vi "Starast.vi"(4 "Ry":i32, 6 "Rx":i32, 8 "Centre Y":i32, 9 "Centre X":i32, 11 "Table Astrometry IN":T1 {"LONGPOLE" format="%.1f"}) -> (3 "Table Astrometry OUT":T1 {"LONGPOLE" format="%.1f"})   [LabVIEW 2019]
uses:
  Globals.vi
panel:
  in  "remove":bool
  in  "add":bool
  in  "Y":i32
  in  "X":i32
  in  "DEC":dbl format="%<%H:%M:%S>t"
  in  "RA":dbl format="%<%H:%M:%S%1u>t"
  in  "calcul":bool
  in  "cancel":bool
  in  "data":string[][](table) caption="Données Astrométriques"
  # "Cette routine permet de recalculer les paramètres du champ et des tables de \nguidage.  Pour ce faire, il faut qu'il y ait 2 ou 3 lignes de données astrométriques.\n\nRemplissez le tableau en centrant une étoile brillante dont la position est connue\nprès du centre optique, puis au moins une deuxième à plus de 15 minutes d'arc\ndu centre.  Idéalement, on voudra en enregistrer une 3e perpendiculairement\nà la deuxième et aussi éloignez d'au moins 15 minutes d'arc des deux autres.\n\nLorsque vous avez terminé, appuyer sur calculer pour voir le résultat du calcul \nou sur annuler pour ignorer tout ce qui a été fait ici."
  # "Voir la possibilité de faire le calcul sur\ntous les couples de 3 coordonnées ..."
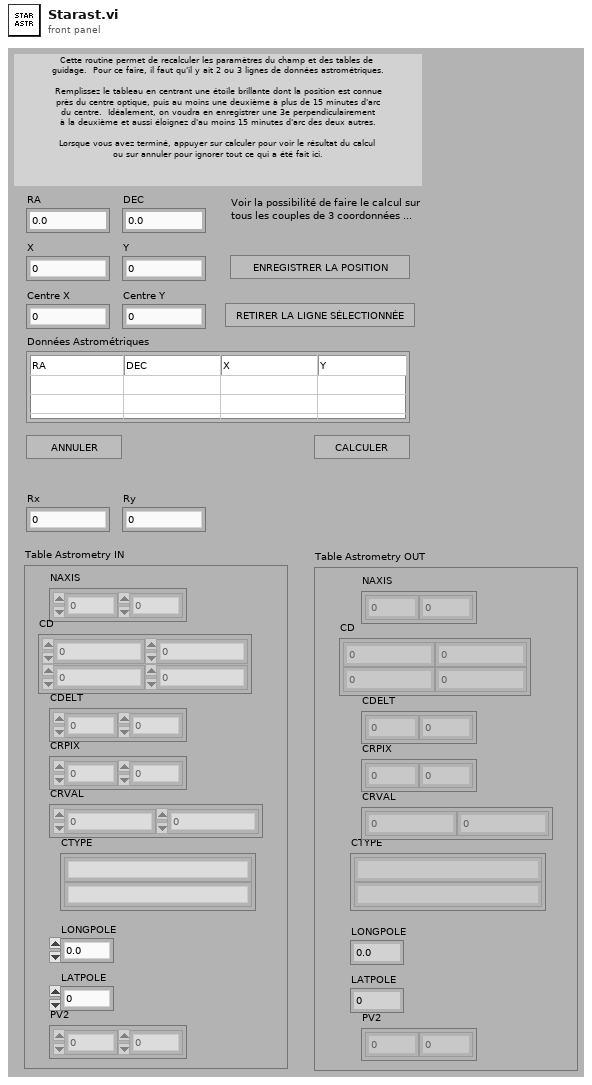
[diagram p1: front panel]
types:
  T1 = cluster{"NAXIS":dbl[], "CD":dbl[][], "CDELT":dbl[], "CRPIX":dbl[], "CTYPE":string[], "CRVAL":dbl[], "LONGPOLE":dbl, "LATPOLE":dbl, "PV2":dbl[]}
  T2 = typedef "LVRowAndColumnTypeDef.ctl" = cluster{"Row":i32, "Column":i32}
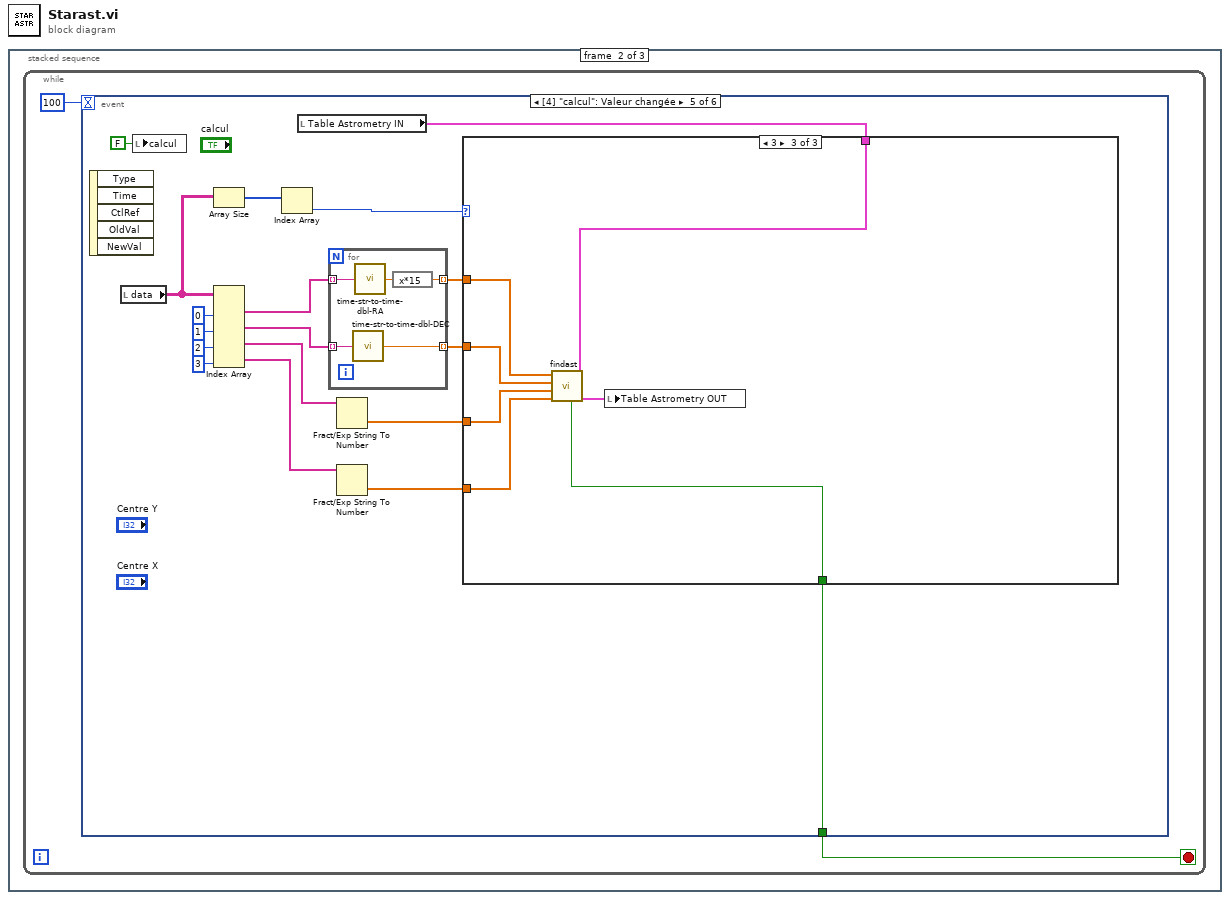
[diagram p0: block diagram]
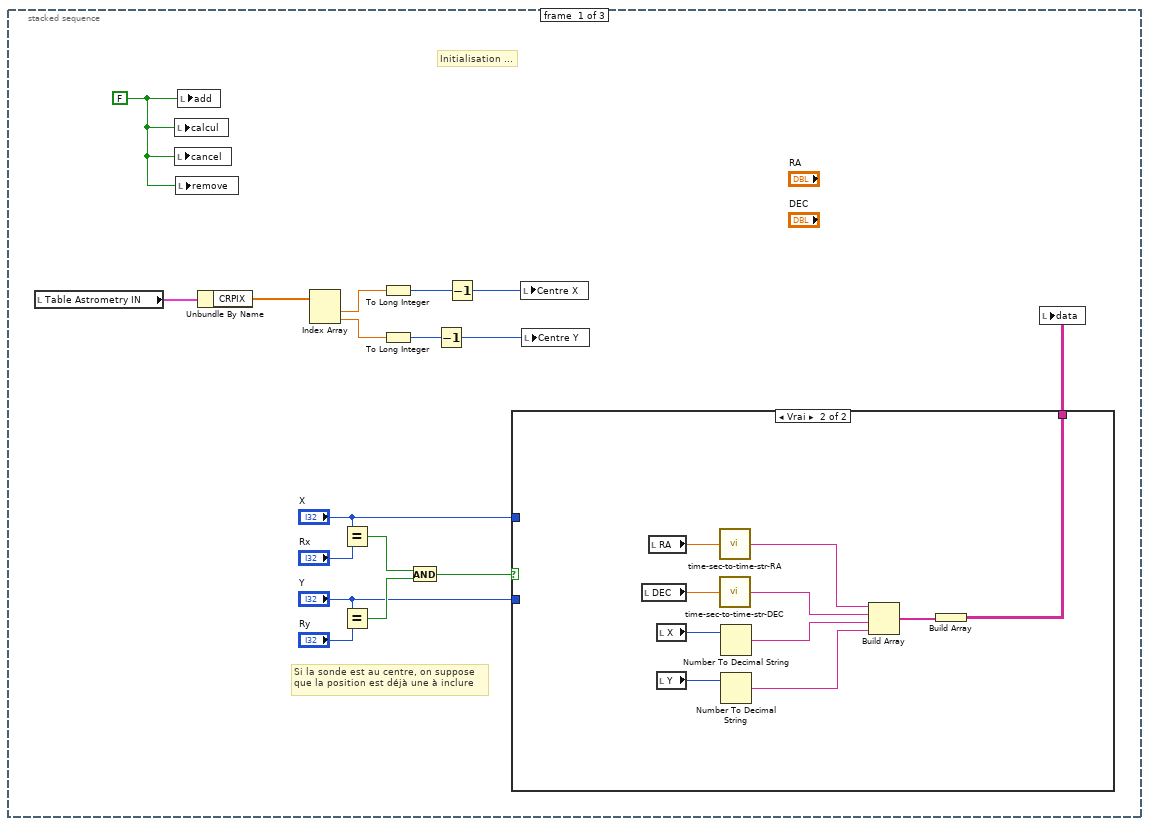
[diagram p2: hidden frame]
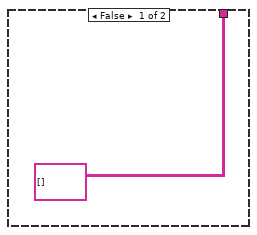
[diagram p3: hidden frame]
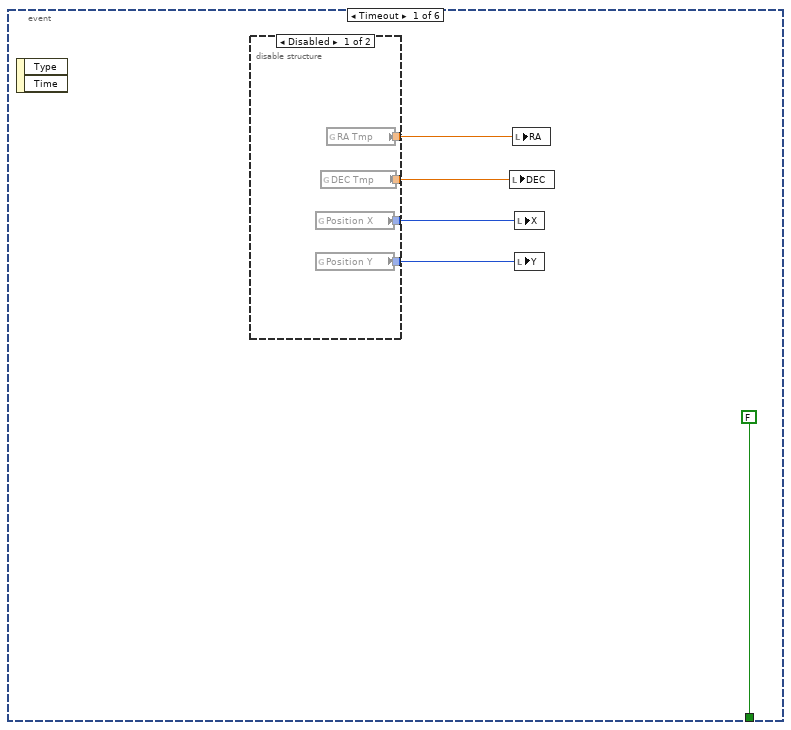
[diagram p4: hidden frame]
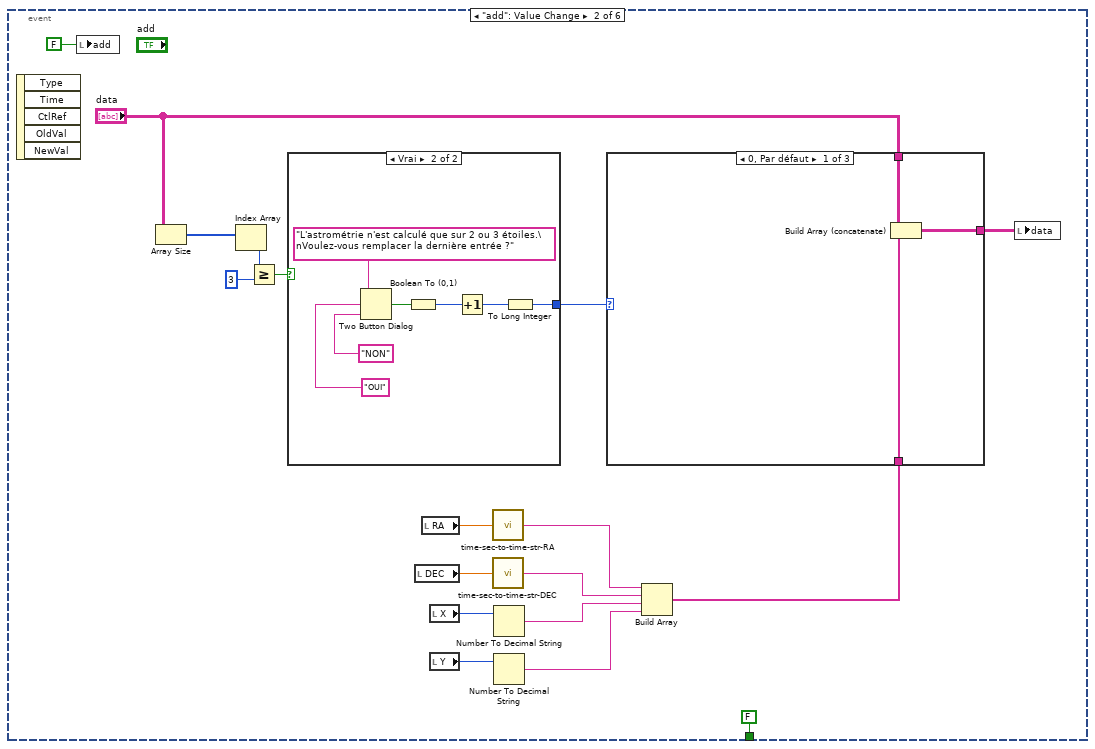
[diagram p6: hidden frame]
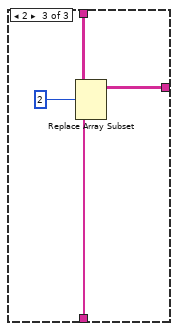
[diagram p8: hidden frame]
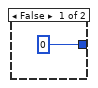
[diagram p9: hidden frame]
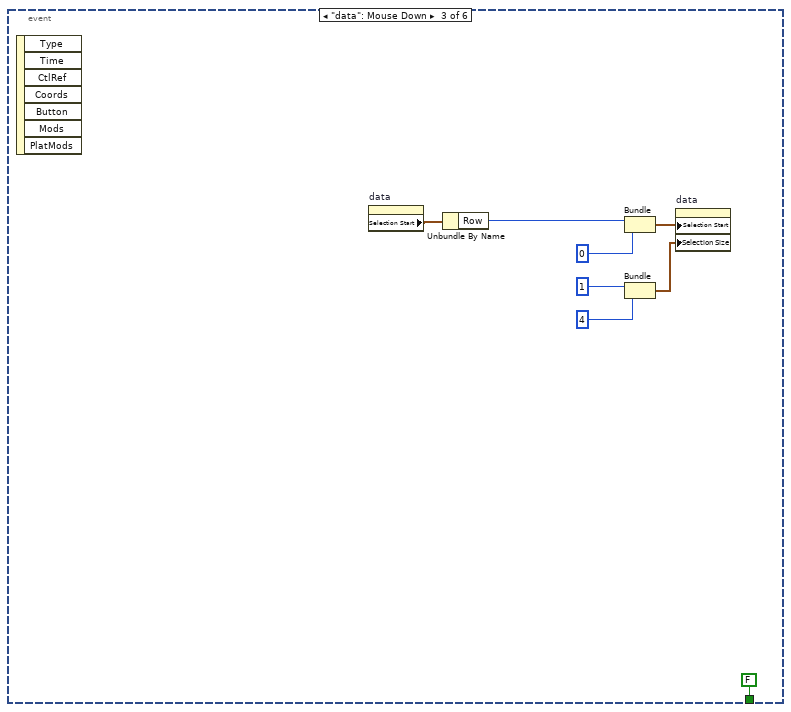
[diagram p10: hidden frame]
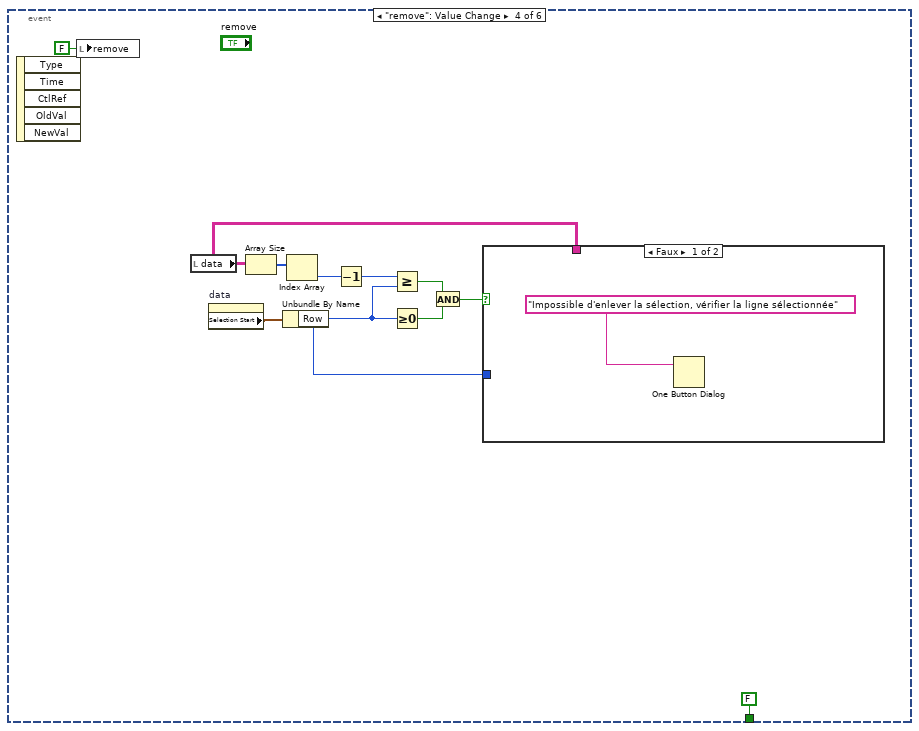
[diagram p11: hidden frame]
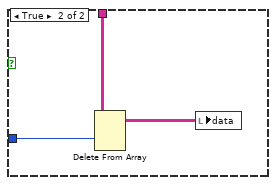
[diagram p12: hidden frame]
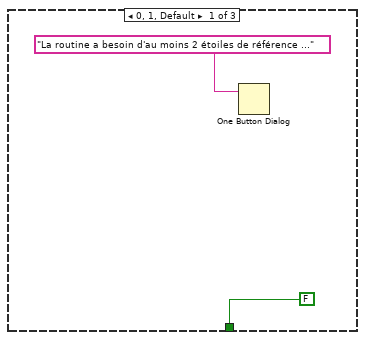
[diagram p13: hidden frame]
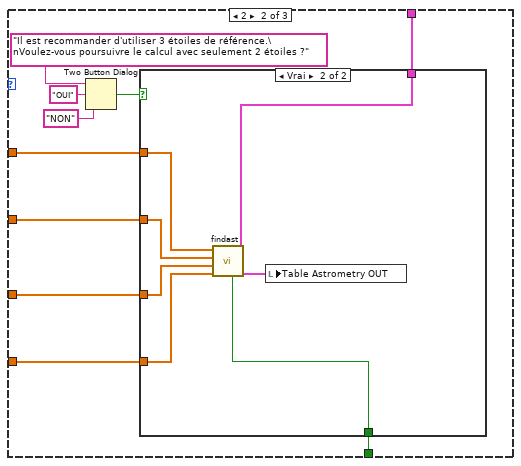
[diagram p14: hidden frame]
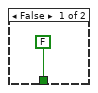
[diagram p15: hidden frame]
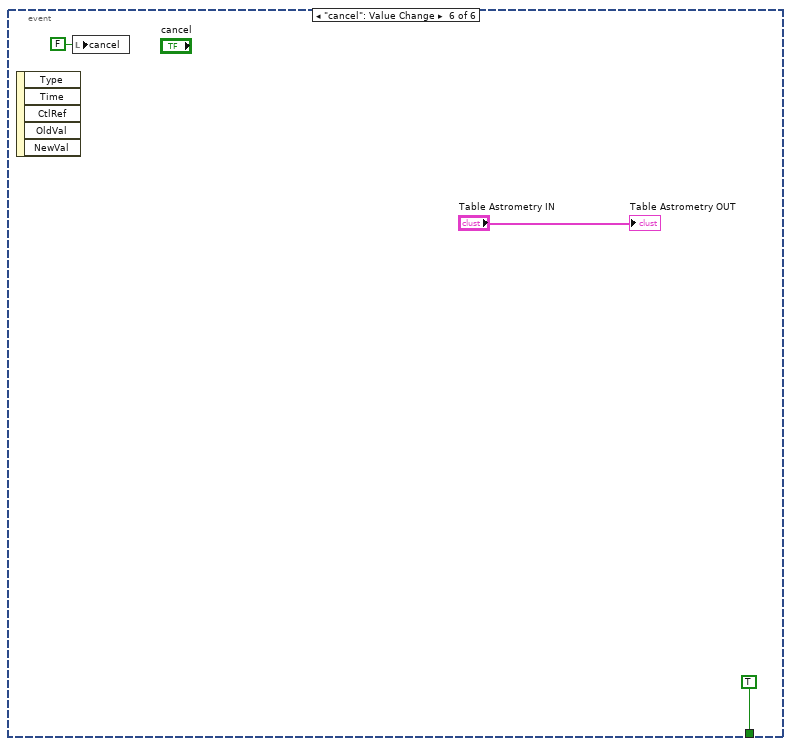
[diagram p16: hidden frame]
diagram:
  n1 = stacked-sequence {
    frame #0 {
      w17 = FALSE ("save")
      # "Si la sonde est au centre, on suppose\nque la position est déjà une à inclure"
      # "Initialisation ..."
      n2 = local read "Table Astrometry IN"() -> (w16:T1)
      n3 = local write "calcul"(w17) -> ()
      n4 = local write "cancel"(w17) -> ()
      n5 = local write "remove"(w17) -> ()
      n6 = local write "add"(w17) -> ()
      n7 = Unbundle By Name(w16) -> ("CRPIX"=w15:dbl[])
      n8 = Index Array(array=w15) -> (element #1=w13:dbl, element #2=w14:dbl)  [unwired: 2 in]
      n9 = Equal?(x="X", y="Rx") -> (x = y?=w8:bool)
      n10 = Equal?(x="Y", y="Ry") -> (x = y?=w7:bool)
      n11 = To Long Integer(number=w13) -> (32bit integer=w12:i32)
      n12 = To Long Integer(number=w14) -> (32bit integer=w11:i32)
      n13 = And(x=w8, y=w7) -> (x .and. y?=w6:bool)
      n14 = Decrement(x=w11) -> (x-1=w1:i32)
      n15 = Decrement(x=w12) -> (x-1=w2:i32)
      n16 = case shown="Vrai" w6 {
        tunnel: [string[][] [] w19] -> w5
        tunnel: "X" -> [_ _]
        tunnel: "Y" -> [_ _]
        frame False {
        }
        frame True {
          n17 = local read "DEC"() -> (w22:dbl)
          n18 = local read "RA"() -> (w21:dbl)
          n19 = local read "X"() -> (w27:i32)
          n20 = local read "Y"() -> (w28:i32)
          n21 = call "time-sec-to-time-str-RA.vi"("Numeric"=w21) -> ("formatted-str"=w23:string)
          n22 = call "time-sec-to-time-str-DEC.vi"("Numeric"=w22) -> ("formatted-str"=w24:string)
          n23 = Number To Decimal String(number=w27) -> (decimal integer string=w25:string)  [unwired: 1 in]
          n24 = Number To Decimal String(number=w28) -> (decimal integer string=w26:string)  [unwired: 1 in]
          n25 = Build Array(w23, w24, w25, w26) -> (w20:string[])
          n26 = Build Array(w20) -> (w19:string[][])
        }
      }
      n27 = local write "Centre X"(w2) -> ()
      n28 = local write "Centre Y"(w1) -> ()
      n29 = local write "data"(w5) -> ()
    }
    frame #1 {
      n30 = while {
        stop <- w30 stop-if-true
        n31 = event shown="[4] \"calcul\": Valeur changée" {
          selector: _ -> [_ _ _ _ _ _]
          dyn-events: _ -> [_ _ _ _ _ _]
          timeout: 100 -> [_ _ _ _ _ _]
          tunnel: [FALSE FALSE FALSE FALSE w108 TRUE] -> w30
          event Timeout {
            n32 = event-data() -> ()  [unwired: 1 in, 2 out]
            n33 = disable-structure shown="Disabled" {
              disable-tunnel: [w39 _] -> w34
              disable-tunnel: [w38 _] -> w33
              disable-tunnel: [w37 _] -> w32
              disable-tunnel: [w36 _] -> w31
              frame Disabled {
                n34 = global read "Globals.vi" "Position X"() -> (w39)
                n35 = global read "Globals.vi" "Position Y"() -> (w38)
                n36 = global read "Globals.vi" "DEC Tmp"() -> (w36:dbl)
                n37 = global read "Globals.vi" "RA Tmp"() -> (w37:dbl)
              }
              frame Enabled {
              }
            }
            n38 = local write "DEC"(w31) -> ()
            n39 = local write "RA"(w32) -> ()
            n40 = local write "X"(w34) -> ()
            n41 = local write "Y"(w33) -> ()
          }
          event "add": Value Change {
            n42 = event-data() -> ()  [unwired: 1 in, 5 out]
            n43 = local write "add"(FALSE) -> ()
            n44 = Array Size(array="data") -> (size(s)=w57:i32[])
            n45 = Index Array(array=w57) -> (element=w54:i32)  [unwired: 1 in]
            n46 = Greater Or Equal?(x=w54, y=3) -> (x >= y?=w55:bool)
            n47 = case shown="Vrai" w55 {
              tunnel: [0 w67] -> w51
              frame False {
              }
              frame True {
                n48 = Two Button Dialog(message="L'astrométrie n'est calculé que sur 2 ou 3 étoiles.\nVoulez-vous remplacer la dernière entrée ?", 1:"NON", 2:"OUI") -> (T button?=w70:bool)
                n49 = Boolean To (0,1)(Boolean=w70) -> (0, 1=w69:i16)
                n50 = Increment(x=w69) -> (x+1=w68:i16)
                n51 = To Long Integer(number=w68) -> (32bit integer=w67:i32)
              }
            }
            n52 = local read "DEC"() -> (w44:dbl)
            n53 = local read "RA"() -> (w43:dbl)
            n54 = local read "X"() -> (w49:i32)
            n55 = local read "Y"() -> (w50:i32)
            n56 = call "time-sec-to-time-str-RA.vi"("Numeric"=w43) -> ("formatted-str"=w45:string)
            n57 = call "time-sec-to-time-str-DEC.vi"("Numeric"=w44) -> ("formatted-str"=w46:string)
            n58 = Number To Decimal String(number=w49) -> (decimal integer string=w47:string)  [unwired: 1 in]
            n59 = Number To Decimal String(number=w50) -> (decimal integer string=w48:string)  [unwired: 1 in]
            n60 = Build Array(w45, w46, w47, w48) -> (w42:string[])
            n61 = case shown="0, Par défaut" w51 {
              tunnel: [w60 w61 w64] -> w53
              tunnel: "data" -> [w59 w61 w65]
              tunnel: w42 -> [w58 _ w63]
              frame 0, Default {
                n62 = Build Array (concatenate)(w59, w58) -> (w60:string[][])
              }
              frame 1 {
              }
              frame 2 {
                n63 = Replace Array Subset(array=w65, new element=w63, index (row)=2) -> (w64:string[][])  [unwired: 1 in]
              }
            }
            n64 = local write "data"(w53) -> ()
          }
          event "data": Mouse Down {
            n65 = event-data() -> ()  [unwired: 1 in, 7 out]
            n66 = property on="data" class="Tbl (strict)"() -> ("Selection Start"=w81:T2)  [unwired: 2 in, 2 out]
            n67 = Unbundle By Name(w81) -> ("Row"=w79:i32)
            n68 = Bundle("Row"=w79, 0) -> (w80:cluster{"Row":i32, i32})  [unwired: 1 in]
            n69 = Bundle(1, 4) -> (w75:cluster{i32, i32})  [unwired: 1 in]
            n70 = property on="data" class="Tbl (strict)"("Selection Start"=w80, "Selection Size"=w75) -> ()  [unwired: 2 in, 2 out]
          }
          event "remove": Value Change {
            n71 = event-data() -> ()  [unwired: 1 in, 5 out]
            n72 = local write "remove"(FALSE ("remove")) -> ()
            n73 = local read "data"() -> (w88:string[][])
            n74 = property on="data" class="Tbl (strict)"() -> ("Selection Start"=w91:T2)  [unwired: 2 in, 2 out]
            n75 = Array Size(array=w88) -> (size(s)=w90:i32[])
            n76 = Unbundle By Name(w91) -> ("Row"=w86:i32)
            n77 = Index Array(array=w90) -> (element=w89:i32)  [unwired: 1 in]
            n78 = Decrement(x=w89) -> (x-1=w87:i32)
            n79 = Greater Or Equal?(x=w87, y=w86) -> (x >= y?=w85:bool)
            n80 = Greater Or Equal To 0?(x=w86) -> (x >= 0?=w84:bool)
            n81 = And(x=w85, y=w84) -> (x .and. y?=w83:bool)
            n82 = case shown="Faux" w83 {
              tunnel: w88 -> [_ w96]
              tunnel: w86 -> [_ w95]
              frame False {
                n83 = One Button Dialog(message="Impossible d'enlever la sélection, vérifier la ligne sélectionnée") -> ()  [unwired: 1 in, 1 out]
              }
              frame True {
                n84 = Delete From Array(array=w96, index (row)=w95) -> (array with subset deleted=w94:string[][])  [unwired: 2 in, 1 out]
                n85 = local write "data"(w94) -> ()
              }
            }
          }
          event "calcul": Value Change {
            n86 = event-data() -> ()  [unwired: 1 in, 5 out]
            n87 = local read "data"() -> (w99:string[][])
            n88 = local write "calcul"(FALSE ("calcul")) -> ()
            n89 = Array Size(array=w99) -> (size(s)=w109:i32[])
            n90 = Index Array(array=w99, index (col) #1=0 ("disabled index (col)"), index (col) #2=1 ("index (col)"), index (col) #3=2 ("index (col)"), index (col) #4=3 ("index (col)")) -> (element #1=w97:string[], element #2=w98:string[], element #3=w106:string[], element #4=w105:string[])  [unwired: 4 in]
            n91 = Index Array(array=w109) -> (element=w107:i32)  [unwired: 1 in]
            n92 = local read "Table Astrometry IN"() -> (w100:T1)
            n93 = for {
              tunnel: w98 -> [w118] mode=indexing
              tunnel: w97 -> [w119] mode=indexing
              tunnel: [w116] -> w104 mode=indexing
              tunnel: [w115] -> w103 mode=indexing
              n94 = call "time-str-to-time-dbl-DEC.vi"("Chaîne"=w118) -> ("TCS_coords"=w115:dbl)
              n95 = call "time-str-to-time-dbl-RA.vi"("Chaîne"=w119) -> ("TCS_coords"=w117:dbl)
              n96 = expression code="x*15"(w117) -> (w116:dbl)
            }
            n97 = Fract/Exp String To Number(string=w106) -> (number=w102:dbl[])  [unwired: 3 in, 1 out]
            n98 = Fract/Exp String To Number(string=w105) -> (number=w101:dbl[])  [unwired: 3 in, 1 out]
            n99 = case shown="3" w107 {
              tunnel: [FALSE w127 w141] -> w108
              tunnel: w104 -> [_ w123 w145]
              tunnel: w103 -> [_ w124 w144]
              tunnel: w102 -> [_ w126 w143]
              tunnel: w101 -> [_ w125 w142]
              tunnel: w100 -> [_ w122 w140]
              frame 0, 1, Default {
                n100 = One Button Dialog(message="La routine a besoin d'au moins 2 étoiles de référence ...") -> ()  [unwired: 1 in, 1 out]
              }
              frame 2 {
                n101 = Two Button Dialog(message="Il est recommander d'utiliser 3 étoiles de référence.\nVoulez-vous poursuivre le calcul avec seulement 2 étoiles ?", 1:"NON" ("F button name (\"Cancel\")"), 2:"OUI" ("T button name (\"OK\")")) -> (T button?=w128:bool)
                n102 = case shown="Vrai" w128 {
                  tunnel: [FALSE w133] -> w127
                  tunnel: w126 -> [_ w137]
                  tunnel: w125 -> [_ w136]
                  tunnel: w124 -> [_ w138]
                  tunnel: w123 -> [_ w139]
                  tunnel: w122 -> [_ w135]
                  frame False {
                  }
                  frame True {
                    n103 = call "findast.vi"("ImgAstrom IN"=w135, "Y"=w136, "X"=w137, "DEC"=w138, "RA"=w139) -> ("ImgAstrom OUT"=w134:T1, "Accepted?"=w133:bool)  [unwired: 5 in]
                    n104 = local write "Table Astrometry OUT"(w134) -> ()
                  }
                }
              }
              frame 3 {
                n105 = call "findast.vi"("ImgAstrom IN"=w140, "Y"=w142, "X"=w143, "DEC"=w144, "RA"=w145) -> ("ImgAstrom OUT"=w146:T1, "Accepted?"=w141:bool)  [unwired: 5 in]
                n106 = local write "Table Astrometry OUT"(w146) -> ()
              }
            }
          }
          event "cancel": Value Change {
            n107 = event-data() -> ()  [unwired: 1 in, 5 out]
            n108 = local write "cancel"(FALSE ("cancel")) -> ()
            "Table Astrometry OUT" <- "Table Astrometry IN"
          }
        }
      }
    }
    frame #2 {
    }
  }
